vi "V550decode.vi"(7 "V550 data":i32[](array[numeric]) format="%.0x") -> (1 "streap":i32[](array[numeric]), 3 "value":i32[](array[numeric]))   [LabVIEW 2014]
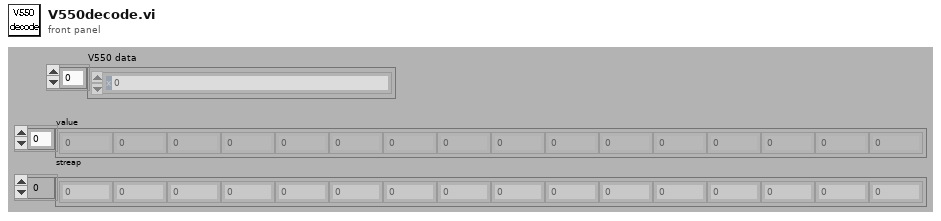
[diagram p1: front panel]
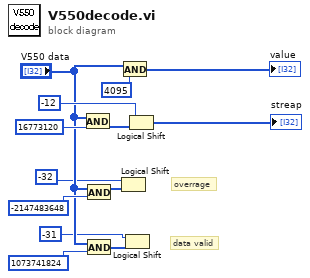
[diagram p0: block diagram]
diagram:
  # "data valid"
  # "overrage"
  n1 = And(x="V550 data", y=16773120) -> (x .and. y?=w10:i32[])
  n2 = And(x="V550 data", y=-2147483648) -> (x .and. y?=w4:i32[])
  n3 = And(x="V550 data", y=1073741824) -> (x .and. y?=w6:i32[])
  n4 = Logical Shift(y=-32, x=w4) -> ()  [unwired: 1 out]
  n5 = And(x="V550 data", y=4095) -> (x .and. y?=→"value":i32[])
  n6 = Logical Shift(y=-31, x=w6) -> ()  [unwired: 1 out]
  n7 = Logical Shift(y=-12, x=w10) -> (x << y=→"streap":i32[])
